vi "DIO_PWM.vi"(0 "DIO.OUT":bool, 1 "DIO.DIR":bool, 6 "DIO/PWM":refnum<k21>="ConnectorA/DIO0") -> (14 "DIO.IN":bool)   [LabVIEW 2019]
doc: "This VI switches between the DIO functionality and the PWM functionality for the specified FPGA I/O channels.\n- If <b>SELECT</b> is FALSE, DIO is enabled.\n- If <b>SELECT</b> is TRUE, PWM is enabled."
panel:
  # "This VI switches between the DIO functionality and the PWM functionality for the specified FPGA I/O channels.\n- If SELECT is FALSE, DIO is enabled.\n- If SELECT is TRUE, PWM is enabled."
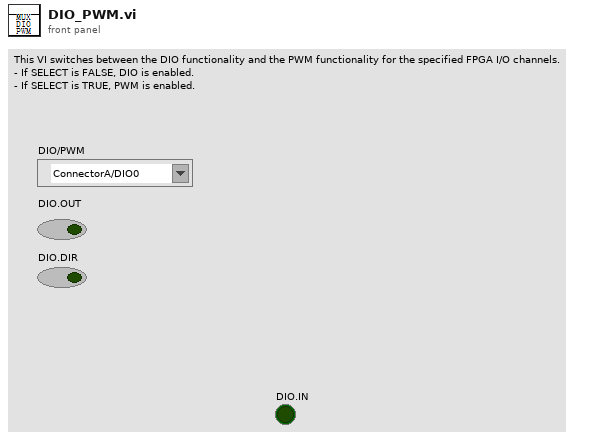
[diagram p1: front panel]
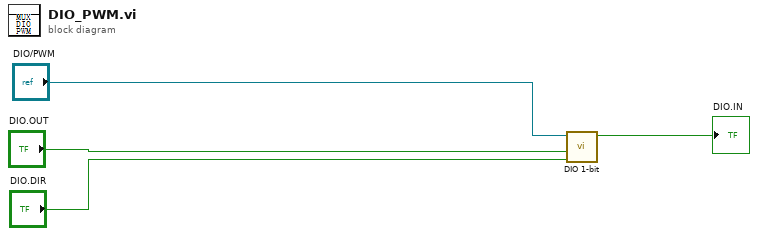
[diagram p0: block diagram]
diagram:
  n1 = call "DIO 1-bit.vi"("DIR"="DIO.DIR", "OUT"="DIO.OUT", "DIO Refnum"="DIO/PWM") -> ("IN"=→"DIO.IN":bool)  [unwired: 8 in]
